vi "Connect.vi"(6 "Network Settings":T2={"Peer IP Address"="localhost"}, 8 "error in (no error)":errorcluster, 9 "timeout in ms (10000)":i32, 10 "General Settings":T3) -> (0 "error out":errorcluster, 3 "Network_Streams out":T1)   [LabVIEW 2020, in "Communication VIs.lvlib" / "Network.lvlib"]
uses:
  Network.lvlib
  Communication/IP_Communication/typedefs/General Settings.ctl
  Communication/IP_Communication/typedefs/Endpoint Tag.ctl
  Network Settings.ctl
  Network Streams.ctl
  Communication/IP_Communication/IP_Communication.lvclass
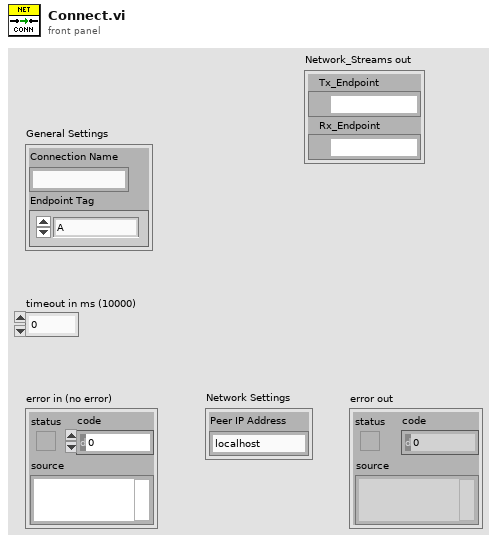
[diagram p1: front panel]
types:
  T1 = typedef "Communication VIs.lvlib/Network.lvlib/Network Streams.ctl" = cluster{"Tx_Endpoint":refnum<k21>, "Rx_Endpoint":refnum<k21>}
  T2 = typedef "Communication VIs.lvlib/Network.lvlib/Network Settings.ctl" = cluster{"Peer IP Address":string}
  T3 = typedef "Communication Classes.lvlib/IP_Communication.lvclass/General Settings.ctl" = cluster{"Connection Name":string, "Endpoint Tag":T4}
  T4 = typedef "Communication Classes.lvlib/IP_Communication.lvclass/Endpoint Tag.ctl" = enum8{"A", "B"}
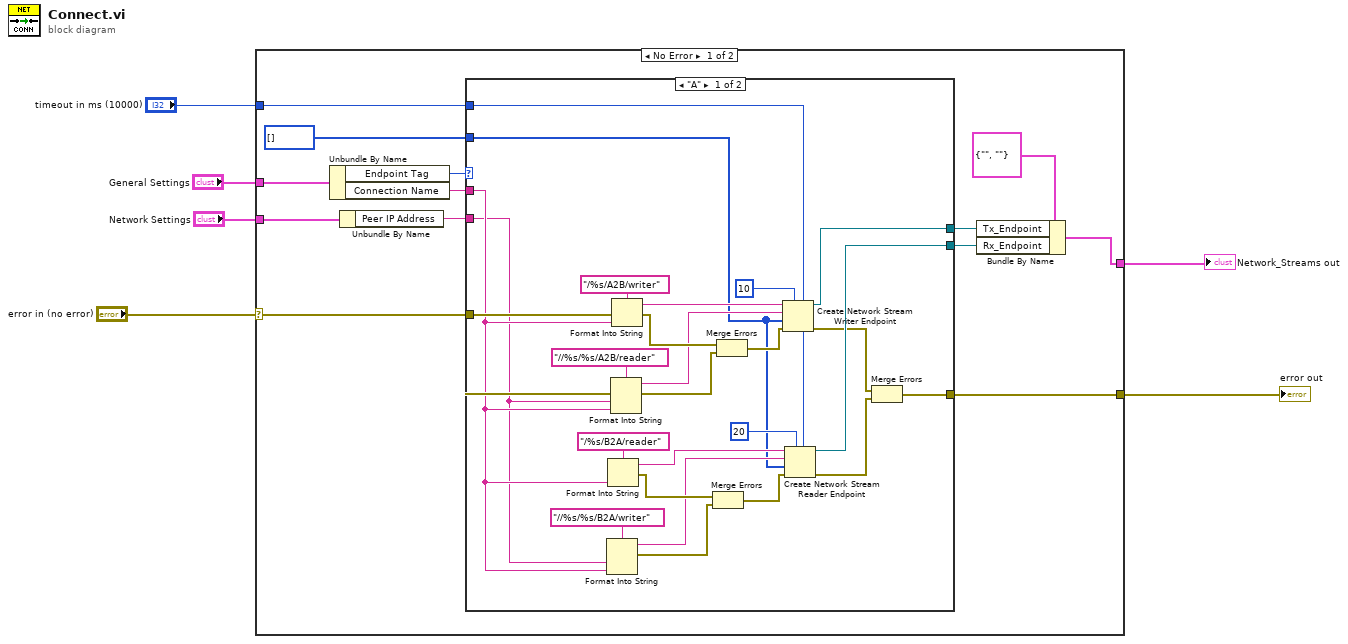
[diagram p0: block diagram]
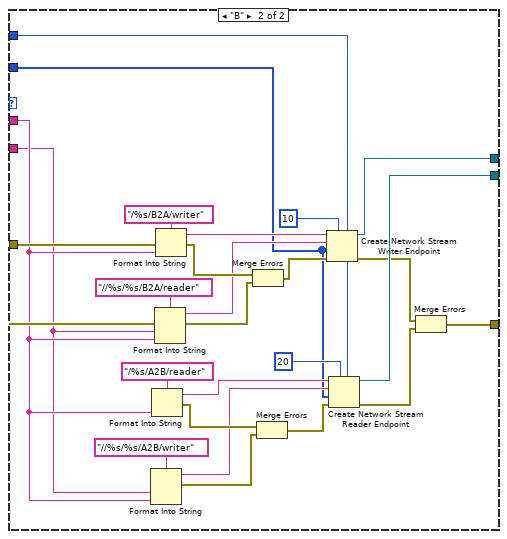
[diagram p2: hidden frame]
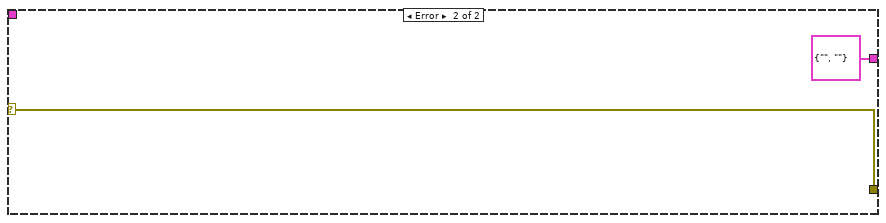
[diagram p3: hidden frame]
diagram:
  n1 = case shown="No Error" "error in (no error)" {
    selector: "error in (no error)" -> [w18 w73]
    tunnel: "Network Settings" -> [w19 _]
    tunnel: "timeout in ms (10000)" -> [w14 _]
    tunnel: [w11 w73] -> w6
    tunnel: [w7 T1 {"Tx_Endpoint"="", "Rx_Endpoint"=""} ("Network_Streams out")] -> w1
    tunnel: "General Settings" -> [w9 _]
    frame No Error {
      n2 = Unbundle By Name(w9) -> ("Endpoint Tag"=w10:T4, "Connection Name"=w16:string)
      n3 = Unbundle By Name(w19) -> ("Peer IP Address"=w15:string)
      n4 = case shown="\"A\"" w10 {
        tunnel: u8[] [] -> [w20 w46]
        tunnel: w18 -> [w32 w58]
        tunnel: w16 -> [w31 w57]
        tunnel: w15 -> [w30 w56]
        tunnel: w14 -> [w26 w52]
        tunnel: [w25 w51] -> w13
        tunnel: [w24 w50] -> w12
        tunnel: [w21 w47] -> w11
        frame "A" {
          n5 = Format Into String(format string="//%s/%s/B2A/writer", w30, w31) -> (resulting string=w28:string, error out=w36:errorcluster)  [unwired: 2 in]
          n6 = Format Into String(format string="/%s/B2A/reader", w31) -> (resulting string=w29:string, error out=w37:errorcluster)  [unwired: 2 in]
          n7 = Format Into String(format string="//%s/%s/A2B/reader", error in=w32, w30, w31) -> (resulting string=w38:string, error out=w40:errorcluster)  [unwired: 1 in]
          n8 = Format Into String(format string="/%s/A2B/writer", error in=w32, w31) -> (resulting string=w44:string, error out=w39:errorcluster)  [unwired: 1 in]
          n9 = Merge Errors(w37, w36) -> (w34:errorcluster)
          n10 = Merge Errors(w39, w40) -> (w41:errorcluster)
          n11 = Create Network Stream Writer Endpoint(5:w26, 7:10 ("writer buffer size"), 8:w41, 9:w20, 10:w38, 11:w44) -> (0:w23:errorcluster, 3:w25:refnum<k21>)  [unwired: 1 in]
          n12 = Create Network Stream Reader Endpoint(5:w26, 7:20 ("reader buffer size"), 8:w34, 9:w20, 10:w28, 11:w29) -> (0:w22:errorcluster, 3:w24:refnum<k21>)  [unwired: 1 in]
          n13 = Merge Errors(w23, w22) -> (w21:errorcluster)
        }
        frame "B" {
          n14 = Format Into String(format string="//%s/%s/A2B/writer", w56, w57) -> (resulting string=w54:string, error out=w62:errorcluster)  [unwired: 2 in]
          n15 = Format Into String(format string="/%s/A2B/reader", w57) -> (resulting string=w55:string, error out=w63:errorcluster)  [unwired: 2 in]
          n16 = Format Into String(format string="//%s/%s/B2A/reader", error in=w58, w56, w57) -> (resulting string=w64:string, error out=w66:errorcluster)  [unwired: 1 in]
          n17 = Format Into String(format string="/%s/B2A/writer", error in=w58, w57) -> (resulting string=w70:string, error out=w65:errorcluster)  [unwired: 1 in]
          n18 = Merge Errors(w65, w66) -> (w67:errorcluster)
          n19 = Merge Errors(w63, w62) -> (w60:errorcluster)
          n20 = Create Network Stream Writer Endpoint(5:w52, 7:10 ("writer buffer size"), 8:w67, 9:w46, 10:w64, 11:w70) -> (0:w49:errorcluster, 3:w51:refnum<k21>)  [unwired: 1 in]
          n21 = Create Network Stream Reader Endpoint(5:w52, 7:20 ("reader buffer size"), 8:w60, 9:w46, 10:w54, 11:w55) -> (0:w48:errorcluster, 3:w50:refnum<k21>)  [unwired: 1 in]
          n22 = Merge Errors(w49, w48) -> (w47:errorcluster)
        }
      }
      n23 = Bundle By Name(cluster=T1 {"Tx_Endpoint"="", "Rx_Endpoint"=""} ("Network_Streams out"), "Tx_Endpoint"=w13, "Rx_Endpoint"=w12) -> (w7:T1)
    }
    frame Error {
    }
  }
  "error out" <- w6
  "Network_Streams out" <- w1
